vi "Dark Current Test Remastered Test Run.vi"() -> ()   [LabVIEW 2020]
uses:
  <vilib>/Utility/file.llb/Write Delimited Spreadsheet (string).vi
  <vilib>/Utility/file.llb/Write Delimited Spreadsheet (DBL).vi
  <instrlib>/CAEN PSM/CAEN PSM.lvlib
panel:
  out "7 4":bool
  out "6 4":bool
  out "8 4":bool
  out "5 4":bool
  out "4 4":bool
  out "3 4":bool
  out "2 4":bool
  out "1 4":bool
  out "Test is Running 4":bool
  out "OVV? 8":bool=TRUE
  out "OVC? 8":bool=TRUE
  out "Actual Voltage Level (V) 8":dbl format="%#_13g"
  out "Actual Current Limit (nA) 4":dbl format="%#_13g"
  in  "dt (s) 4":i32
  out "Time Left (s) 4":dbl
  out "Power Supply Trip 4":bool
  in  "N 4":i32
  in  "Channel # 4":i32
  in  "VISA resource name 4":refnum<visa-resource-name>
  out "OVV? 7":bool=TRUE
  out "OVC? 7":bool=TRUE
  out "Actual Voltage Level (V) 7":dbl format="%#_13g"
  out "Recorded Current\nfor Previous Tube 4":dbl format="%#_13g"
  in  "Measure Next Tube 4":bool
  out "Next Measurment 4":string
  in  "Barcodes 4":string[](array[string])
  out "Manual Measurments \nNeeded 4":bool
  in  "Begin Test 4":bool
  out "7 3":bool
  out "6 3":bool
  out "8 3":bool
  out "5 3":bool
  out "4 3":bool
  out "3 3":bool
  out "2 3":bool
  out "1 3":bool
  out "Test is Running 3":bool
  out "OVV? 6":bool=TRUE
  out "OVC? 6":bool=TRUE
  out "Actual Voltage Level (V) 6":dbl format="%#_13g"
  out "Actual Current Limit (nA) 3":dbl format="%#_13g"
  in  "dt (s) 3":i32
  out "Time Left (s) 3":dbl
  out "Power Supply Trip 3":bool
  in  "N 3":i32
  in  "Channel # 3":i32
  in  "VISA resource name 3":refnum<visa-resource-name>
  out "OVV? 5":bool=TRUE
  out "OVC? 5":bool=TRUE
  out "Actual Voltage Level (V) 5":dbl format="%#_13g"
  out "Recorded Current\nfor Previous Tube 3":dbl format="%#_13g"
  in  "Measure Next Tube 3":bool
  out "Next Measurment 3":string
  in  "Barcodes 3":string[](array[string])
  out "Manual Measurments \nNeeded 3":bool
  in  "Begin Test 3":bool
  out "7 2":bool
  out "6 2":bool
  out "8 2":bool
  out "5 2":bool
  out "4 2":bool
  out "3 2":bool
  out "2 2":bool
  out "1 2":bool
  out "Test is Running 2":bool
  out "OVV? 4":bool=TRUE
  out "OVC? 4":bool=TRUE
  out "Actual Voltage Level (V) 4":dbl format="%#_13g"
  out "Actual Current Limit (nA) 2":dbl format="%#_13g"
  in  "dt (s) 2":i32
  out "Time Left (s) 2":dbl
  out "Power Supply Trip 2":bool
  in  "N 2":i32
  in  "Channel # 2":i32
  in  "VISA resource name 2":refnum<visa-resource-name>
  out "OVV? 3":bool=TRUE
  out "OVC? 3":bool=TRUE
  out "Actual Voltage Level (V) 3":dbl format="%#_13g"
  out "Recorded Current\nfor Previous Tube 2":dbl format="%#_13g"
  in  "Measure Next Tube 2":bool
  out "Next Measurment 2":string
  in  "Barcodes 2":string[](array[string])
  out "Manual Measurments \nNeeded 2":bool
  in  "Begin Test 2":bool
  out "Power Supply Trip":bool
  out "Time Left (s)":dbl
  out "8":bool
  out "7":bool
  out "6":bool
  out "5":bool
  out "4":bool
  out "3":bool
  out "2":bool
  out "1":bool
  out "Test is Running":bool
  in  "Begin Test":bool
  out "Manual Measurments \nNeeded":bool
  out "OVV? 2":bool=TRUE
  out "OVC? 2":bool=TRUE
  out "Actual Voltage Level (V) 2":dbl format="%#_13g"
  out "Recorded Current\nfor Previous Tube":dbl format="%#_13g"
  in  "Measure Next Tube":bool
  in  "Barcodes":string[](array[string])
  out "Next Measurment":string
  in  "N":i32
  in  "dt (s)":i32
  out "Actual Current Limit (nA)":dbl format="%#_13g"
  out "Actual Voltage Level (V)":dbl format="%#_13g"
  out "OVC?":bool=TRUE
  out "OVV?":bool=TRUE
  in  "Channel #":i32
  in  "VISA resource name":refnum<visa-resource-name>
  # "Dark Current Test"
  # "Instructions in Brief:\n1. Begin the program by clicking the white arrow.\n2. Assemble tubes into the test bench.\n3. Select COM5 for the \"VISA resource name\".\n4. Enter in how often you want to take measurement in the \"dt\" box (typically 60s)\n5. Enter in how many measurments you want to take (typically 15)\n6. Scan in the 8 tubes that you are testing.\n(If you take 15 measurments every 60s, the test will take 15 min.)\n7. Click \"Begin Test\". The \"Test is Running\" LED should light up.\n8. After the intial test, if the total current is below 16nA, \n    the program will write the \n     file and end the test.\n9. If the total current is above 16nA, manual\n    measurments need to be taken.\n10. Engage only the tube indicated by \"Next Measurment\". \n11. Click \"Measure\".\n12. Engage the next tube and continue untill all have been measured.\n13. In both cases, the program will write files and end the test. \n14. The test is over when the \"Test is Running\" LED has turned off."
  # "Green lights indicate tubes that have passed."
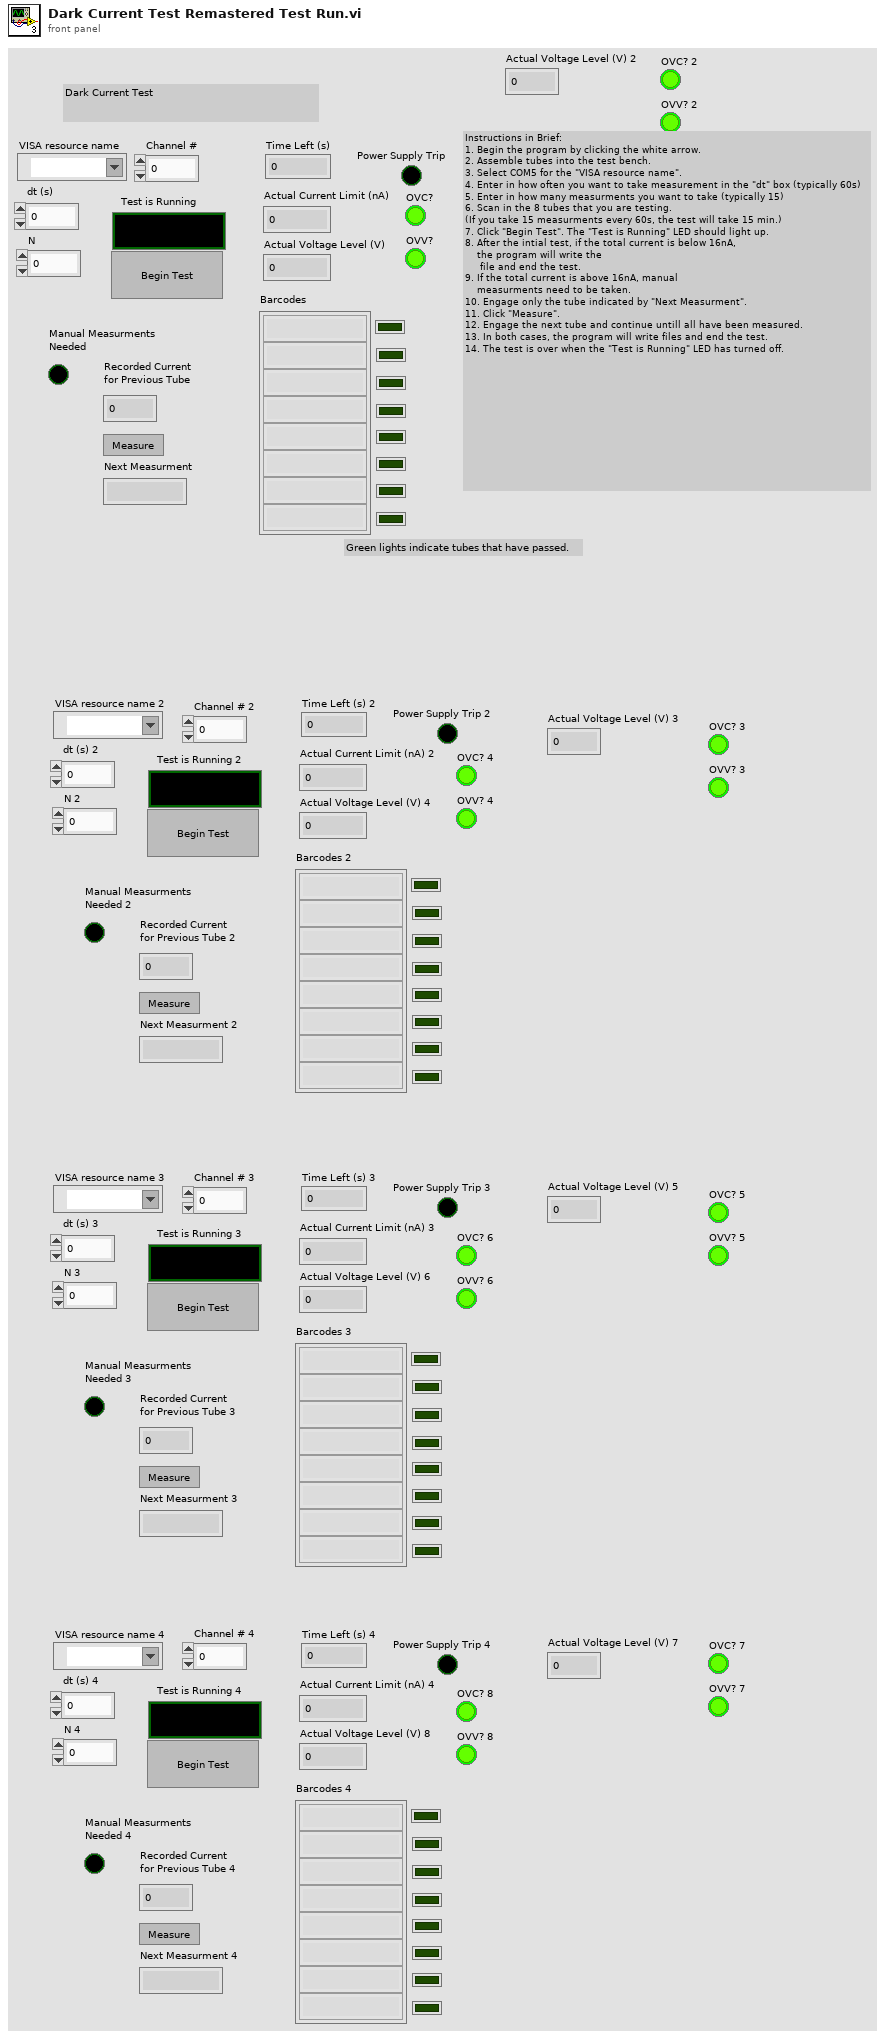
[diagram p1: front panel]
types:
  T1 = cluster{"VISA resource name":refnum<visa-resource-name>, "Board address":u8, "NChannels":u8}
  T2 = cluster{"ON":bool, "RUP":bool, "RDW":bool, "OVC":bool, "OVV":bool, "UNV":bool, "MAXV":bool, "TRIP":bool, "OVP":bool, "OVT":bool, "DIS":bool, "KILL":bool, "ILK":bool, "NOCAL":bool}[]
  T3 = cluster{"ON":bool, "RUP":bool, "RDW":bool, "OVC":bool, "OVV":bool, "UNV":bool, "MAXV":bool, "TRIP":bool, "OVP":bool, "OVT":bool, "DIS":bool, "KILL":bool, "ILK":bool, "NOCAL":bool}
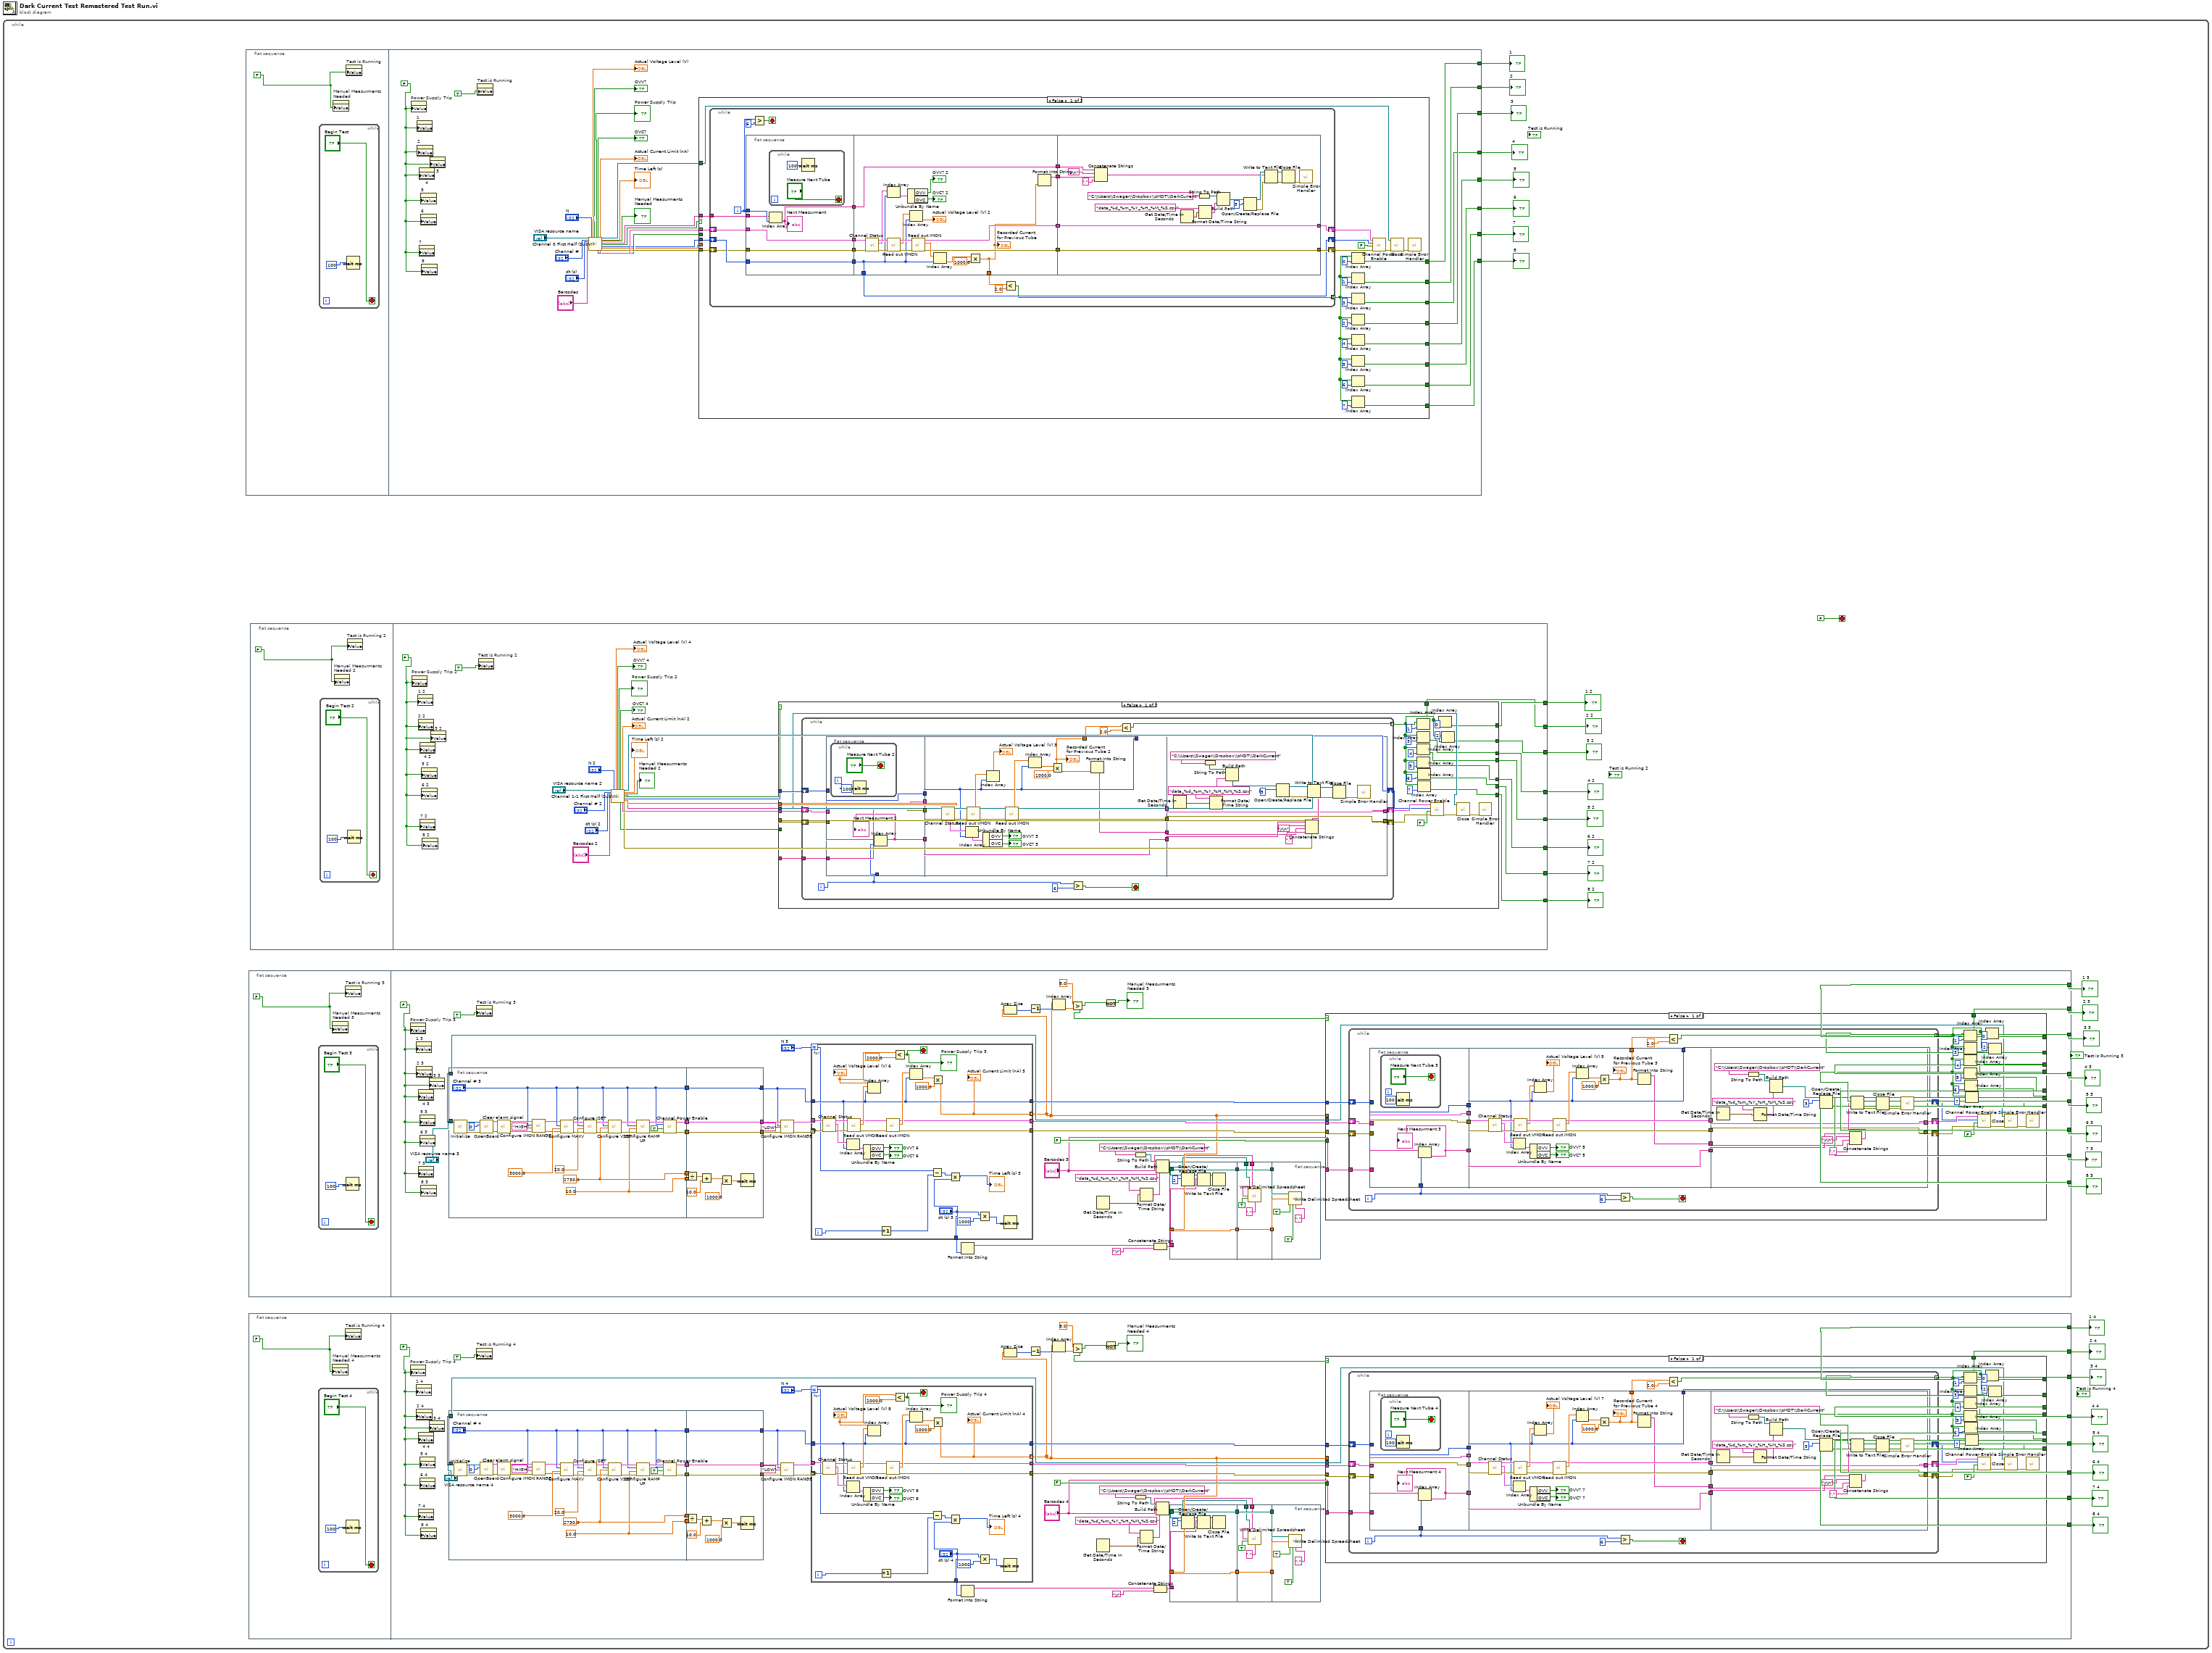
[diagram p0: block diagram]
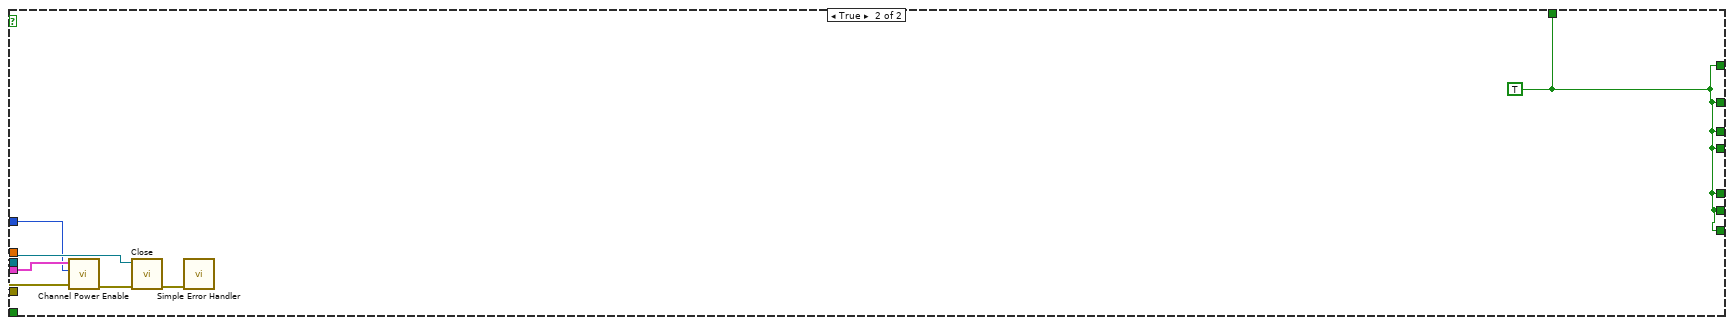
[diagram p2: hidden frame]
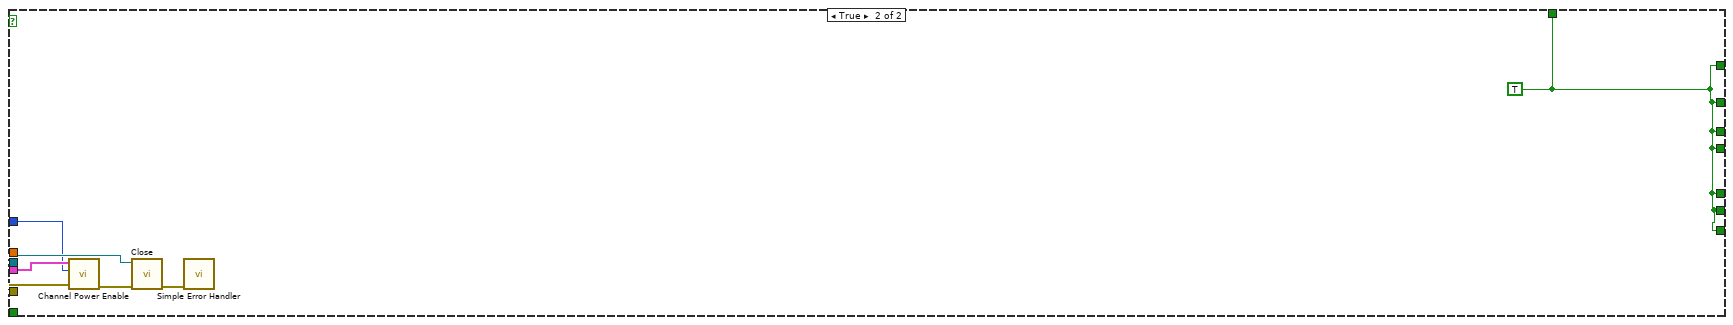
[diagram p3: hidden frame]
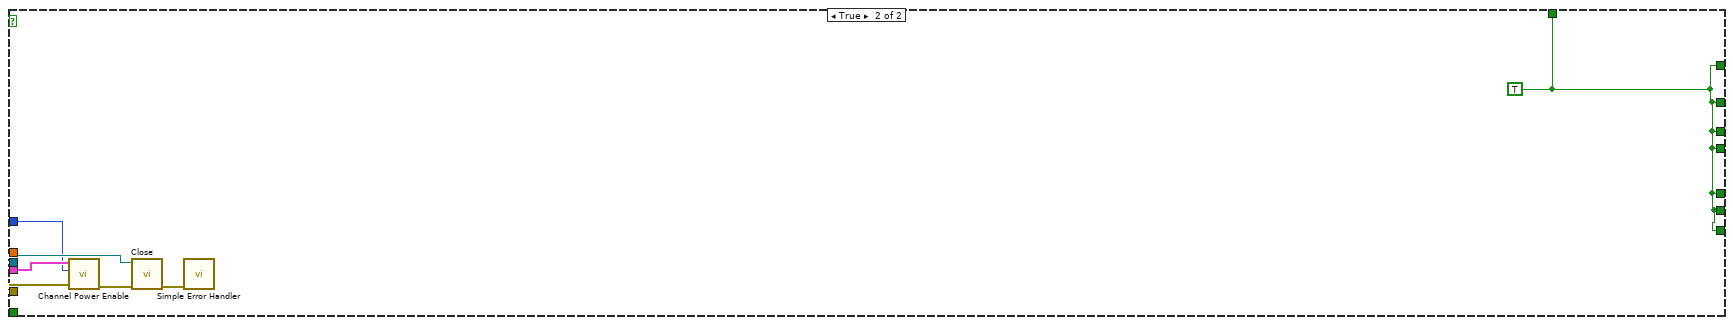
[diagram p4: hidden frame]
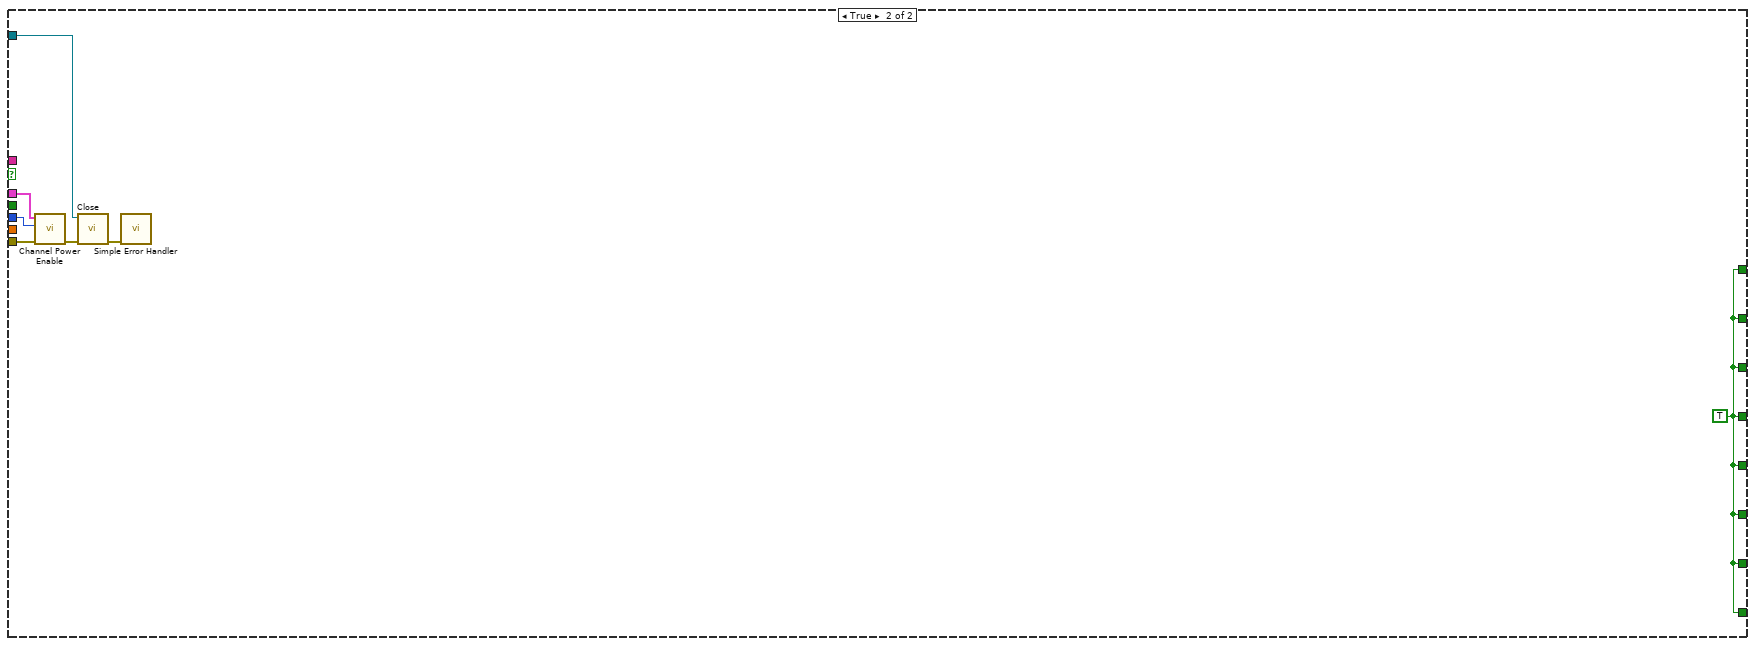
[diagram p5: hidden frame]
diagram:
  n1 = while {
    stop <- FALSE stop-if-true
    n2 = flat-sequence {
      tunnel: [w678] -> w32
      tunnel: [w658] -> w31
      tunnel: [w677] -> w30
      tunnel: [w676] -> w29
      tunnel: [w675] -> w28
      tunnel: [w659] -> w27
      tunnel: [w674] -> w26
      tunnel: [w673] -> w25
      frame #0 {
        w655 = FALSE
        n3 = while {
          stop <- "Begin Test" stop-if-true
          n4 = Wait (ms)(milliseconds to wait=100) -> ()  [unwired: 1 out]
        }
        n5 = property on="Manual Measurments \nNeeded" class="Bool (strict)"("Value"=w655) -> ()  [unwired: 2 in, 2 out]
        n6 = property on="Test is Running" class="Bool (strict)"("Value"=w655) -> ()  [unwired: 2 in, 2 out]
      }
      frame #1 {
        w671 = FALSE
        n7 = property on="Power Supply Trip" class="Bool (strict)"("Value"=w671) -> ()  [unwired: 2 in, 2 out]
        n8 = property on="1" class="Bool (strict)"("Value"=w671) -> ()  [unwired: 2 in, 2 out]
        n9 = property on="2" class="Bool (strict)"("Value"=w671) -> ()  [unwired: 2 in, 2 out]
        n10 = property on="4" class="Bool (strict)"("Value"=w671) -> ()  [unwired: 2 in, 2 out]
        n11 = property on="7" class="Bool (strict)"("Value"=w671) -> ()  [unwired: 2 in, 2 out]
        n12 = property on="5" class="Bool (strict)"("Value"=w671) -> ()  [unwired: 2 in, 2 out]
        n13 = property on="6" class="Bool (strict)"("Value"=w671) -> ()  [unwired: 2 in, 2 out]
        n14 = property on="8" class="Bool (strict)"("Value"=w671) -> ()  [unwired: 2 in, 2 out]
        n15 = property on="3" class="Bool (strict)"("Value"=w671) -> ()  [unwired: 2 in, 2 out]
        n16 = property on="Test is Running" class="Bool (strict)"("Value"=TRUE) -> ()  [unwired: 2 in, 2 out]
        n17 = call "Channel 0 First Half (SubVI).vi"("VISA Refnum in"="VISA resource name", "Channel #"="Channel #", "dt (s)"="dt (s)", "Barcodes in"="Barcodes", "N"="N") -> ("Actual Voltage Level (V)"=→"Actual Voltage Level (V)":dbl, "OVV?"=→"OVV?":bool, "Power Supply Trip"=→"Power Supply Trip":bool, "OVC?"=→"OVC?":bool, "Boolean 2"=w684:bool, "Actual Current Limit (nA)"=→"Actual Current Limit (nA)":dbl, "BoardHandle out 2"=w686:T1, "VISA Refnum out"=w682:refnum<visa-resource-name>, "Time Left (s)"=→"Time Left (s)":dbl, "Manual Measurments \nNeeded"=→"Manual Measurments \nNeeded":bool, "Barcodes out"=w670:string[], "Boolean"=w680:bool, "Channel # out 2"=w683:i32, "Array"=w672:dbl[], "error out"=w685:errorcluster)  [unwired: 8 in]
        n18 = case shown="False" w680 {
          tunnel: w686 -> [w714 w787]
          tunnel: w685 -> [w715 w786]
          tunnel: w684 -> [_ _]
          tunnel: w683 -> [w713 w785]
          tunnel: w682 -> [w709 w788]
          tunnel: w672 -> [_ _]
          tunnel: w670 -> [w705 _]
          tunnel: [w695 w791] -> w678
          tunnel: [w694 w791] -> w658
          tunnel: [w693 w791] -> w677
          tunnel: [w692 w791] -> w676
          tunnel: [w691 w791] -> w675
          tunnel: [w690 w791] -> w659
          tunnel: [w689 w791] -> w674
          tunnel: [w688 w791] -> w673
          frame False {
            n19 = while {
              shift-right: [w721] -> w706
              shift-left: w713 -> [w731]
              shift-right: [w723] -> w708
              shift-left: w714 -> [w728]
              shift-right: [w722] -> w707
              shift-left: w715 -> [w726]
              tunnel: w705 -> [w719]
              tunnel: [w716] -> w704 mode=indexing
              i -> [w734]
              stop <- w735 stop-if-true
              n20 = flat-sequence {
                tunnel: w734 -> [w742]
                tunnel: [w741] -> w733
                tunnel: w731 -> [w740]
                tunnel: [w740] -> w730
                tunnel: [w739] -> w729
                tunnel: w728 -> [w739]
                tunnel: [w738] -> w727
                tunnel: w726 -> [w738]
                tunnel: w719 -> [w737]
                tunnel: w733 -> [w752]
                tunnel: [w752] -> w732
                tunnel: w730 -> [w747]
                tunnel: w729 -> [w750]
                tunnel: w727 -> [w751]
                tunnel: [w749] -> w725
                tunnel: [w748] -> w724
                tunnel: [w747] -> w721
                tunnel: [w746] -> w720
                tunnel: [w745] -> w718
                tunnel: w732 -> [w770]
                tunnel: w725 -> [w768]
                tunnel: w724 -> [w767]
                tunnel: [w768] -> w723
                tunnel: [w767] -> w722
                tunnel: w720 -> [w766]
                frame #0 {
                  n21 = while {
                    stop <- "Measure Next Tube" stop-if-true
                    n22 = Wait (ms)(milliseconds to wait=100) -> ()  [unwired: 1 out]
                  }
                  n23 = Index Array(array=w737, index=w742) -> (element=w741:string)
                  "Next Measurment" <- w741
                }
                frame #1 {
                  n24 = call <instrlib>:"Channel Status.vi"("error in (no error)"=w751, "BoardHandle"=w750) -> ("error out"=w758:errorcluster, "Channel Status Array"=w754:T2, "BoardHandle out"=w759:T1)  [unwired: 7 in]
                  n25 = Index Array(array=w754, index=w747) -> (element=w755:T3)
                  n26 = call <instrlib>:"Read out VMON.vi"("error in (no error)"=w758, "BoardHandle"=w759) -> ("error out"=w762:errorcluster, "VMon values (V)"=w760:dbl[], "BoardHandle out"=w761:T1)  [unwired: 7 in]
                  n27 = Unbundle By Name(w755) -> ("OVV"=→"OVV? 2":bool, "OVC"=→"OVC? 2":bool)
                  n28 = Index Array(array=w760, index=w747) -> (element=→"Actual Voltage Level (V) 2":dbl)
                  n29 = call <instrlib>:"Read out IMON.vi"("error in (no error)"=w762, "BoardHandle"=w761) -> ("error out"=w748:errorcluster, "IMon values (uA)"=w765:dbl[], "BoardHandle out"=w749:T1)  [unwired: 6 in, 1 out]
                  n30 = Index Array(array=w765, index=w747) -> (element=w763:dbl)
                  n31 = Multiply(x=w763, y=1000.0) -> (x*y=w745:dbl)
                  "Recorded Current\nfor Previous Tube" <- w745
                  n32 = Format Into String(w745) -> (resulting string=w746:string)  [unwired: 3 in, 1 out]
                }
                frame #2 {
                  n33 = Concatenate Strings(w770, "\r\n", w766, ",") -> (w772:string)
                  n34 = Get Date/Time In Seconds() -> (seconds since 1Jan1904=w782:timestamp)
                  n35 = String To Path(string="C:\\Users\\Swager\\Dropbox\\sMDT\\DarkCurrent") -> (path=w781:path)
                  n36 = Format Date/Time String(time format string (%c)="data_%d_%m_%Y_%H_%M_%S.csv", seconds (now)=w782) -> (date/time string=w783:string)  [unwired: 1 in]
                  n37 = Build Path(base path=w781, name or relative path=w783) -> (appended path=w779:path)
                  n38 = Open/Create/Replace File(file path (use dialog)=w779, operation (0:open)=5) -> (refnum out=w778:refnum<file>, error out=w777:errorcluster)  [unwired: 4 in, 1 out]
                  n39 = Write to Text File(file (use dialog)=w778, text=w772, error in=w777) -> (refnum out=w776:refnum<file>, error out=w775:errorcluster)  [unwired: 1 in, 1 out]
                  n40 = Close File(refnum=w776, error in=w775) -> (error out=w774:errorcluster)  [unwired: 1 out]
                  n41 = call <vilib>:"Simple Error Handler.vi"("error in (no error)"=w774) -> ()  [unwired: 4 in, 5 out]
                }
              }
              n42 = Greater?(x=w734, y=6) -> (0:w735:bool)
              n43 = Less?(x=w718, y=2.0) -> (x < y?=w716:bool)
            }
            n44 = Index Array(array=w704, index=0) -> (element=w695:bool)
            n45 = Index Array(array=w704, index=1) -> (element=w694:bool)
            n46 = Index Array(array=w704, index=3) -> (element=w692:bool)
            n47 = Index Array(array=w704, index=2) -> (element=w693:bool)
            n48 = Index Array(array=w704, index=4) -> (element=w691:bool)
            n49 = Index Array(array=w704, index=5) -> (element=w690:bool)
            n50 = Index Array(array=w704, index=6) -> (element=w689:bool)
            n51 = Index Array(array=w704, index=7) -> (element=w688:bool)
            n52 = call <instrlib>:"Channel Power Enable.vi"("error in (no error)"=w707, "Enable (OFF)"=FALSE, "Channel (0)"=w706, "BoardHandle"=w708) -> ("error out"=w711:errorcluster)  [unwired: 6 in, 1 out]
            n53 = call <instrlib>:"Close.vi"("error in (no error)"=w711, "VISA resource name"=w709) -> ("error out"=w710:errorcluster)  [unwired: 9 in]
            n54 = call <vilib>:"Simple Error Handler.vi"("error in (no error)"=w710) -> ()  [unwired: 4 in, 5 out]
          }
          frame True {
            w791 = TRUE
            n55 = call <instrlib>:"Channel Power Enable.vi"("error in (no error)"=w786, "Channel (0)"=w785, "BoardHandle"=w787) -> ("error out"=w790:errorcluster)  [unwired: 7 in, 1 out]
            n56 = call <instrlib>:"Close.vi"("error in (no error)"=w790, "VISA resource name"=w788) -> ("error out"=w789:errorcluster)  [unwired: 9 in]
            n57 = call <vilib>:"Simple Error Handler.vi"("error in (no error)"=w789) -> ()  [unwired: 4 in, 5 out]
          }
        }
      }
    }
    n58 = flat-sequence {
      tunnel: [w303] -> w16
      tunnel: [w302] -> w15
      tunnel: [w301] -> w14
      tunnel: [w300] -> w13
      tunnel: [w299] -> w12
      tunnel: [w298] -> w11
      tunnel: [w297] -> w10
      tunnel: [w296] -> w9
      frame #0 {
        w276 = FALSE
        n59 = while {
          stop <- "Begin Test 3" stop-if-true
          n60 = Wait (ms)(milliseconds to wait=100) -> ()  [unwired: 1 out]
        }
        n61 = property on="Manual Measurments \nNeeded 3" class="Bool (strict)"("Value"=w276) -> ()  [unwired: 2 in, 2 out]
        n62 = property on="Test is Running 3" class="Bool (strict)"("Value"=w276) -> ()  [unwired: 2 in, 2 out]
      }
      frame #1 {
        w289 = FALSE
        n63 = property on="Power Supply Trip 3" class="Bool (strict)"("Value"=w289) -> ()  [unwired: 2 in, 2 out]
        n64 = property on="1 3" class="Bool (strict)"("Value"=w289) -> ()  [unwired: 2 in, 2 out]
        n65 = property on="2 3" class="Bool (strict)"("Value"=w289) -> ()  [unwired: 2 in, 2 out]
        n66 = property on="4 3" class="Bool (strict)"("Value"=w289) -> ()  [unwired: 2 in, 2 out]
        n67 = property on="7 3" class="Bool (strict)"("Value"=w289) -> ()  [unwired: 2 in, 2 out]
        n68 = property on="5 3" class="Bool (strict)"("Value"=w289) -> ()  [unwired: 2 in, 2 out]
        n69 = property on="6 3" class="Bool (strict)"("Value"=w289) -> ()  [unwired: 2 in, 2 out]
        n70 = property on="8 3" class="Bool (strict)"("Value"=w289) -> ()  [unwired: 2 in, 2 out]
        n71 = property on="3 3" class="Bool (strict)"("Value"=w289) -> ()  [unwired: 2 in, 2 out]
        n72 = flat-sequence {
          tunnel: [w463] -> w328
          tunnel: [w462] -> w327
          tunnel: [w459] -> w318
          tunnel: [w461] -> w326
          tunnel: [w460] -> w325
          tunnel: ["Channel # 3"] -> w324
          tunnel: "VISA resource name 3" -> [w459]
          tunnel: w328 -> [w483]
          tunnel: w327 -> [w482]
          tunnel: [w481] -> w315
          tunnel: w326 -> [w481]
          tunnel: [w480] -> w316
          tunnel: w325 -> [w480]
          tunnel: [w479] -> w313
          tunnel: w324 -> [w479]
          frame #0 {
            w463 = 2730.0 ("Voltage Set (Volts)")
            w462 = 10.0 ("Voltage Ramp Up (V/s)")
            n73 = call <instrlib>:"Initialize.vi"("VISA resource name"=w459) -> ("error out"=w473:errorcluster, "VISA resource name out"=w469:refnum<visa-resource-name>)  [unwired: 9 in]
            n74 = call <instrlib>:"OpenBoard.vi"("error in (no error)"=w473, "Board Address"=0, "VISA resource name"=w469) -> ("error out"=w474:errorcluster, "BoardHandle"=w468:T1)  [unwired: 7 in]
            n75 = call <instrlib>:"Clear alarm signal.vi"("error in (no error)"=w474, "BoardHandle"=w468) -> ("error out"=w457:errorcluster, "BoardHandle out"=w456:T1)  [unwired: 8 in]
            n76 = call <instrlib>:"Configure IMON RANGE.vi"("error in (no error)"=w457, "IMon range (LOW)"="HIGH", "Channel (0)"="Channel # 3", "BoardHandle"=w456) -> ("error out"=w452:errorcluster, "BoardHandle out"=w453:T1)  [unwired: 6 in]
            n77 = call <instrlib>:"Configure MAXV.vi"("error in (no error)"=w452, "Voltage Max (0.0 V)"=3000.0 ("VMax (Volts)"), "Channel (0)"="Channel # 3", "BoardHandle"=w453) -> ("error out"=w475:errorcluster, "BoardHandle out"=w467:T1)  [unwired: 6 in]
            n78 = call <instrlib>:"Configure ISET.vi"("error in (no error)"=w475, "Current Limit (0.00 uA)"=20.0 ("Current Limit (uA)"), "Channel (0)"="Channel # 3", "BoardHandle"=w467) -> ("error out"=w476:errorcluster, "BoardHandle out"=w466:T1)  [unwired: 6 in]
            n79 = call <instrlib>:"Configure VSET.vi"("error in (no error)"=w476, "Voltage Level (0.0 V)"=w463, "Channel (0)"="Channel # 3", "BoardHandle"=w466) -> ("error out"=w477:errorcluster, "BoardHandle out"=w465:T1)  [unwired: 6 in]
            n80 = call <instrlib>:"Configure RAMP UP.vi"("error in (no error)"=w477, "Voltage ramp up (0 V/s)"=w462, "Channel (0)"="Channel # 3", "BoardHandle"=w465) -> ("error out"=w478:errorcluster, "BoardHandle out"=w464:T1)  [unwired: 6 in]
            n81 = call <instrlib>:"Channel Power Enable.vi"("error in (no error)"=w478, "Enable (OFF)"=TRUE ("Boolean"), "Channel (0)"="Channel # 3", "BoardHandle"=w464) -> ("error out"=w460:errorcluster, "BoardHandle out"=w461:T1)  [unwired: 6 in]
          }
          frame #1 {
            n82 = Divide(x=w483, y=w482) -> (x/y=w486:dbl)
            n83 = Add(x=w486, y=10.0) -> (x+y=w487:dbl)
            n84 = Multiply(x=w487, y=1000.0) -> (x*y=w488:dbl)
            n85 = Wait (ms)(milliseconds to wait=w488) -> ()  [unwired: 1 out]
          }
        }
        n86 = property on="Test is Running 3" class="Bool (strict)"("Value"=TRUE) -> ()  [unwired: 2 in, 2 out]
        n87 = call <instrlib>:"Configure IMON RANGE.vi"("error in (no error)"=w316, "IMon range (LOW)"="LOW", "Channel (0)"=w313, "BoardHandle"=w315) -> ("error out"=w311:errorcluster, "BoardHandle out"=w312:T1)  [unwired: 6 in]
        n88 = for {
          N: "N 3" -> [w497]
          tunnel: w311 -> [w504]
          tunnel: w313 -> [w505]
          tunnel: [w507] -> w322
          tunnel: [w506] -> w321
          tunnel: [w498] -> w290 mode=indexing
          tunnel: [w505] -> w319
          tunnel: w312 -> [w501]
          tunnel: [w504] -> _ mode=indexing
          tunnel: ["dt (s) 3"] -> w288
          i -> [w494]
          stop <- w492 stop-if-true
          n89 = call <instrlib>:"Channel Status.vi"("error in (no error)"=w504, "BoardHandle"=w501) -> ("error out"=w513:errorcluster, "Channel Status Array"=w517:T2, "BoardHandle out"=w512:T1)  [unwired: 7 in]
          n90 = Index Array(array=w517, index=w505) -> (element=w516:T3)
          n91 = call <instrlib>:"Read out VMON.vi"("error in (no error)"=w513, "BoardHandle"=w512) -> ("error out"=w509:errorcluster, "VMon values (V)"=w511:dbl[], "BoardHandle out"=w510:T1)  [unwired: 7 in]
          n92 = Unbundle By Name(w516) -> ("OVV"=→"OVV? 6":bool, "OVC"=→"OVC? 6":bool)
          n93 = Index Array(array=w511, index=w505) -> (element=w491:dbl)
          "Actual Voltage Level (V) 6" <- w491
          n94 = Increment(x=w494) -> (x+1=w493:i32)
          n95 = call <instrlib>:"Read out IMON.vi"("error in (no error)"=w509, "BoardHandle"=w510) -> ("error out"=w506:errorcluster, "IMon values (uA)"=w508:dbl[], "BoardHandle out"=w507:T1)  [unwired: 6 in, 1 out]
          n96 = Less?(x=w491, y=2000.0) -> (x < y?=w492:bool)
          "Power Supply Trip 3" <- w492
          n97 = Index Array(array=w508, index=w505) -> (element=w500:dbl)
          n98 = Subtract(x=w497, y=w493) -> (x-y=w496:i32)
          n99 = Multiply(x=w500, y=1000.0) -> (x*y=w498:dbl)
          "Actual Current Limit (nA) 3" <- w498
          n100 = Multiply(x=w496, y="dt (s) 3") -> (x*y=→"Time Left (s) 3":i32)
          n101 = Multiply(x="dt (s) 3", y=1000) -> (x*y=w503:i32)
          n102 = Wait (ms)(milliseconds to wait=w503) -> ()  [unwired: 1 out]
        }
        n103 = Format Into String(w288) -> (resulting string=w280:string)  [unwired: 3 in, 1 out]
        n104 = Array Size(array=w290) -> (size(s)=w310:i32)
        n105 = Decrement(x=w310) -> (x-1=w309:i32)
        n106 = Index Array(array=w290, index=w309) -> (element=w308:dbl)
        n107 = Greater?(x=8.0, y=w308) -> (0:w307:bool)
        n108 = Get Date/Time In Seconds() -> (seconds since 1Jan1904=w293:timestamp)
        n109 = Not(x=w307) -> (.not. x?=→"Manual Measurments \nNeeded 3":bool)
        n110 = String To Path(string="C:\\Users\\Swager\\Dropbox\\sMDT\\DarkCurrent") -> (path=w292:path)
        n111 = Format Date/Time String(time format string (%c)="data_%d_%m_%Y_%H_%M_%S.csv", seconds (now)=w293) -> (date/time string=w294:string)  [unwired: 1 in]
        n112 = Concatenate Strings(w280, "\r") -> (w281:string)
        n113 = Build Path(base path=w292, name or relative path=w294) -> (appended path=w283:path)
        n114 = flat-sequence {
          tunnel: w283 -> [w335]
          tunnel: [w335] -> w287
          tunnel: [w336] -> w285
          tunnel: w290 -> [w336]
          tunnel: w281 -> [w332]
          tunnel: w287 -> [w342]
          tunnel: [w342] -> w286
          tunnel: w285 -> [w341]
          tunnel: [w341] -> w284
          tunnel: w283 -> [w340]
          tunnel: "Barcodes 3" -> [w339]
          tunnel: w286 -> [w345]
          tunnel: w284 -> [w344]
          frame #0 {
            n115 = Open/Create/Replace File(file path (use dialog)=w335, operation (0:open)=2) -> (refnum out=w333:refnum<file>, error out=w334:errorcluster)  [unwired: 4 in, 1 out]
            n116 = Write to Text File(file (use dialog)=w333, text=w332, error in=w334) -> (refnum out=w330:refnum<file>, error out=w331:errorcluster)  [unwired: 1 in, 1 out]
            n117 = Close File(refnum=w330, error in=w331) -> ()  [unwired: 2 out]
          }
          frame #1 {
            n118 = call-poly <vilib>:"Write Delimited Spreadsheet.vi"("file path (dialog if empty)"=w340, "1D data"=w339, "append to file? (new file:F)"=TRUE, "delimiter (\\t)"=",") -> ()  [unwired: 10 in, 2 out]
          }
          frame #2 {
            n119 = call-poly <vilib>:"Write Delimited Spreadsheet.vi"("file path (dialog if empty)"=w345, "1D data"=w344, "append to file? (new file:F)"=TRUE, "transpose? (no:F)"=TRUE, "delimiter (\\t)"=",") -> ()  [unwired: 9 in, 2 out]
          }
        }
        n120 = case shown="False" w307 {
          tunnel: w322 -> [w374 w447]
          tunnel: w321 -> [w375 w446]
          tunnel: FALSE -> [_ _]
          tunnel: w319 -> [w373 w445]
          tunnel: w318 -> [w369 w448]
          tunnel: w290 -> [_ _]
          tunnel: "Barcodes 3" -> [w365 _]
          tunnel: [w355 w451] -> w303
          tunnel: [w354 w451] -> w302
          tunnel: [w353 w451] -> w301
          tunnel: [w352 w451] -> w300
          tunnel: [w351 w451] -> w299
          tunnel: [w350 w451] -> w298
          tunnel: [w349 w451] -> w297
          tunnel: [w348 w451] -> w296
          frame False {
            n121 = while {
              shift-right: [w381] -> w366
              shift-left: w373 -> [w391]
              shift-right: [w383] -> w368
              shift-left: w374 -> [w388]
              shift-right: [w382] -> w367
              shift-left: w375 -> [w386]
              tunnel: w365 -> [w379]
              tunnel: [w376] -> w364 mode=indexing
              i -> [w394]
              stop <- w395 stop-if-true
              n122 = flat-sequence {
                tunnel: w394 -> [w402]
                tunnel: [w401] -> w393
                tunnel: w391 -> [w400]
                tunnel: [w400] -> w390
                tunnel: [w399] -> w389
                tunnel: w388 -> [w399]
                tunnel: [w398] -> w387
                tunnel: w386 -> [w398]
                tunnel: w379 -> [w397]
                tunnel: w393 -> [w412]
                tunnel: [w412] -> w392
                tunnel: w390 -> [w407]
                tunnel: w389 -> [w410]
                tunnel: w387 -> [w411]
                tunnel: [w409] -> w385
                tunnel: [w408] -> w384
                tunnel: [w407] -> w381
                tunnel: [w406] -> w380
                tunnel: [w405] -> w378
                tunnel: w392 -> [w430]
                tunnel: w385 -> [w428]
                tunnel: w384 -> [w427]
                tunnel: [w428] -> w383
                tunnel: [w427] -> w382
                tunnel: w380 -> [w426]
                frame #0 {
                  n123 = while {
                    stop <- "Measure Next Tube 3" stop-if-true
                    n124 = Wait (ms)(milliseconds to wait=100) -> ()  [unwired: 1 out]
                  }
                  n125 = Index Array(array=w397, index=w402) -> (element=w401:string)
                  "Next Measurment 3" <- w401
                }
                frame #1 {
                  n126 = call <instrlib>:"Channel Status.vi"("error in (no error)"=w411, "BoardHandle"=w410) -> ("error out"=w418:errorcluster, "Channel Status Array"=w414:T2, "BoardHandle out"=w419:T1)  [unwired: 7 in]
                  n127 = Index Array(array=w414, index=w407) -> (element=w415:T3)
                  n128 = call <instrlib>:"Read out VMON.vi"("error in (no error)"=w418, "BoardHandle"=w419) -> ("error out"=w422:errorcluster, "VMon values (V)"=w420:dbl[], "BoardHandle out"=w421:T1)  [unwired: 7 in]
                  n129 = Unbundle By Name(w415) -> ("OVV"=→"OVV? 5":bool, "OVC"=→"OVC? 5":bool)
                  n130 = Index Array(array=w420, index=w407) -> (element=→"Actual Voltage Level (V) 5":dbl)
                  n131 = call <instrlib>:"Read out IMON.vi"("error in (no error)"=w422, "BoardHandle"=w421) -> ("error out"=w408:errorcluster, "IMon values (uA)"=w425:dbl[], "BoardHandle out"=w409:T1)  [unwired: 6 in, 1 out]
                  n132 = Index Array(array=w425, index=w407) -> (element=w423:dbl)
                  n133 = Multiply(x=w423, y=1000.0) -> (x*y=w405:dbl)
                  "Recorded Current\nfor Previous Tube 3" <- w405
                  n134 = Format Into String(w405) -> (resulting string=w406:string)  [unwired: 3 in, 1 out]
                }
                frame #2 {
                  n135 = Get Date/Time In Seconds() -> (seconds since 1Jan1904=w442:timestamp)
                  n136 = String To Path(string="C:\\Users\\Swager\\Dropbox\\sMDT\\DarkCurrent") -> (path=w441:path)
                  n137 = Format Date/Time String(time format string (%c)="data_%d_%m_%Y_%H_%M_%S.csv", seconds (now)=w442) -> (date/time string=w443:string)  [unwired: 1 in]
                  n138 = Build Path(base path=w441, name or relative path=w443) -> (appended path=w439:path)
                  n139 = Open/Create/Replace File(file path (use dialog)=w439, operation (0:open)=5) -> (refnum out=w438:refnum<file>, error out=w437:errorcluster)  [unwired: 4 in, 1 out]
                  n140 = Concatenate Strings(w430, "\r\n", w426, ",") -> (w432:string)
                  n141 = Write to Text File(file (use dialog)=w438, text=w432, error in=w437) -> (refnum out=w436:refnum<file>, error out=w435:errorcluster)  [unwired: 1 in, 1 out]
                  n142 = Close File(refnum=w436, error in=w435) -> (error out=w434:errorcluster)  [unwired: 1 out]
                  n143 = call <vilib>:"Simple Error Handler.vi"("error in (no error)"=w434) -> ()  [unwired: 4 in, 5 out]
                }
              }
              n144 = Greater?(x=w394, y=6) -> (0:w395:bool)
              n145 = Less?(x=w378, y=2.0) -> (x < y?=w376:bool)
            }
            n146 = Index Array(array=w364, index=1) -> (element=w354:bool)
            n147 = Index Array(array=w364, index=3) -> (element=w352:bool)
            n148 = Index Array(array=w364, index=4) -> (element=w351:bool)
            n149 = Index Array(array=w364, index=5) -> (element=w350:bool)
            n150 = Index Array(array=w364, index=6) -> (element=w349:bool)
            n151 = Index Array(array=w364, index=7) -> (element=w348:bool)
            n152 = call <instrlib>:"Channel Power Enable.vi"("error in (no error)"=w367, "Enable (OFF)"=FALSE, "Channel (0)"=w366, "BoardHandle"=w368) -> ("error out"=w371:errorcluster)  [unwired: 6 in, 1 out]
            n153 = Index Array(array=w364, index=0) -> (element=w355:bool)
            n154 = Index Array(array=w364, index=2) -> (element=w353:bool)
            n155 = call <instrlib>:"Close.vi"("error in (no error)"=w371, "VISA resource name"=w369) -> ("error out"=w370:errorcluster)  [unwired: 9 in]
            n156 = call <vilib>:"Simple Error Handler.vi"("error in (no error)"=w370) -> ()  [unwired: 4 in, 5 out]
          }
          frame True {
            w451 = TRUE
            n157 = call <instrlib>:"Channel Power Enable.vi"("error in (no error)"=w446, "Channel (0)"=w445, "BoardHandle"=w447) -> ("error out"=w450:errorcluster)  [unwired: 7 in, 1 out]
            n158 = call <instrlib>:"Close.vi"("error in (no error)"=w450, "VISA resource name"=w448) -> ("error out"=w449:errorcluster)  [unwired: 9 in]
            n159 = call <vilib>:"Simple Error Handler.vi"("error in (no error)"=w449) -> ()  [unwired: 4 in, 5 out]
          }
        }
      }
    }
    n160 = flat-sequence {
      tunnel: [w61] -> w8
      tunnel: [w60] -> w7
      tunnel: [w59] -> w6
      tunnel: [w58] -> w5
      tunnel: [w57] -> w4
      tunnel: [w56] -> w3
      tunnel: [w55] -> w2
      tunnel: [w54] -> w1
      frame #0 {
        w34 = FALSE
        n161 = while {
          stop <- "Begin Test 4" stop-if-true
          n162 = Wait (ms)(milliseconds to wait=100) -> ()  [unwired: 1 out]
        }
        n163 = property on="Manual Measurments \nNeeded 4" class="Bool (strict)"("Value"=w34) -> ()  [unwired: 2 in, 2 out]
        n164 = property on="Test is Running 4" class="Bool (strict)"("Value"=w34) -> ()  [unwired: 2 in, 2 out]
      }
      frame #1 {
        w47 = FALSE
        n165 = property on="Power Supply Trip 4" class="Bool (strict)"("Value"=w47) -> ()  [unwired: 2 in, 2 out]
        n166 = property on="1 4" class="Bool (strict)"("Value"=w47) -> ()  [unwired: 2 in, 2 out]
        n167 = property on="2 4" class="Bool (strict)"("Value"=w47) -> ()  [unwired: 2 in, 2 out]
        n168 = property on="4 4" class="Bool (strict)"("Value"=w47) -> ()  [unwired: 2 in, 2 out]
        n169 = property on="7 4" class="Bool (strict)"("Value"=w47) -> ()  [unwired: 2 in, 2 out]
        n170 = property on="5 4" class="Bool (strict)"("Value"=w47) -> ()  [unwired: 2 in, 2 out]
        n171 = property on="6 4" class="Bool (strict)"("Value"=w47) -> ()  [unwired: 2 in, 2 out]
        n172 = property on="8 4" class="Bool (strict)"("Value"=w47) -> ()  [unwired: 2 in, 2 out]
        n173 = property on="3 4" class="Bool (strict)"("Value"=w47) -> ()  [unwired: 2 in, 2 out]
        n174 = flat-sequence {
          tunnel: [w221] -> w86
          tunnel: [w220] -> w85
          tunnel: [w217] -> w76
          tunnel: [w219] -> w84
          tunnel: [w218] -> w83
          tunnel: ["Channel # 4"] -> w82
          tunnel: "VISA resource name 4" -> [w217]
          tunnel: w86 -> [w241]
          tunnel: w85 -> [w240]
          tunnel: [w239] -> w73
          tunnel: w84 -> [w239]
          tunnel: [w238] -> w74
          tunnel: w83 -> [w238]
          tunnel: [w237] -> w71
          tunnel: w82 -> [w237]
          frame #0 {
            w221 = 2730.0 ("Voltage Set (Volts)")
            w220 = 10.0 ("Voltage Ramp Up (V/s)")
            n175 = call <instrlib>:"Initialize.vi"("VISA resource name"=w217) -> ("error out"=w231:errorcluster, "VISA resource name out"=w227:refnum<visa-resource-name>)  [unwired: 9 in]
            n176 = call <instrlib>:"OpenBoard.vi"("error in (no error)"=w231, "Board Address"=0, "VISA resource name"=w227) -> ("error out"=w232:errorcluster, "BoardHandle"=w226:T1)  [unwired: 7 in]
            n177 = call <instrlib>:"Clear alarm signal.vi"("error in (no error)"=w232, "BoardHandle"=w226) -> ("error out"=w215:errorcluster, "BoardHandle out"=w214:T1)  [unwired: 8 in]
            n178 = call <instrlib>:"Configure IMON RANGE.vi"("error in (no error)"=w215, "IMon range (LOW)"="HIGH", "Channel (0)"="Channel # 4", "BoardHandle"=w214) -> ("error out"=w210:errorcluster, "BoardHandle out"=w211:T1)  [unwired: 6 in]
            n179 = call <instrlib>:"Configure MAXV.vi"("error in (no error)"=w210, "Voltage Max (0.0 V)"=3000.0 ("VMax (Volts)"), "Channel (0)"="Channel # 4", "BoardHandle"=w211) -> ("error out"=w233:errorcluster, "BoardHandle out"=w225:T1)  [unwired: 6 in]
            n180 = call <instrlib>:"Configure ISET.vi"("error in (no error)"=w233, "Current Limit (0.00 uA)"=20.0 ("Current Limit (uA)"), "Channel (0)"="Channel # 4", "BoardHandle"=w225) -> ("error out"=w234:errorcluster, "BoardHandle out"=w224:T1)  [unwired: 6 in]
            n181 = call <instrlib>:"Configure VSET.vi"("error in (no error)"=w234, "Voltage Level (0.0 V)"=w221, "Channel (0)"="Channel # 4", "BoardHandle"=w224) -> ("error out"=w235:errorcluster, "BoardHandle out"=w223:T1)  [unwired: 6 in]
            n182 = call <instrlib>:"Configure RAMP UP.vi"("error in (no error)"=w235, "Voltage ramp up (0 V/s)"=w220, "Channel (0)"="Channel # 4", "BoardHandle"=w223) -> ("error out"=w236:errorcluster, "BoardHandle out"=w222:T1)  [unwired: 6 in]
            n183 = call <instrlib>:"Channel Power Enable.vi"("error in (no error)"=w236, "Enable (OFF)"=TRUE ("Boolean"), "Channel (0)"="Channel # 4", "BoardHandle"=w222) -> ("error out"=w218:errorcluster, "BoardHandle out"=w219:T1)  [unwired: 6 in]
          }
          frame #1 {
            n184 = Divide(x=w241, y=w240) -> (x/y=w244:dbl)
            n185 = Add(x=w244, y=10.0) -> (x+y=w245:dbl)
            n186 = Multiply(x=w245, y=1000.0) -> (x*y=w246:dbl)
            n187 = Wait (ms)(milliseconds to wait=w246) -> ()  [unwired: 1 out]
          }
        }
        n188 = property on="Test is Running 4" class="Bool (strict)"("Value"=TRUE) -> ()  [unwired: 2 in, 2 out]
        n189 = call <instrlib>:"Configure IMON RANGE.vi"("error in (no error)"=w74, "IMon range (LOW)"="LOW", "Channel (0)"=w71, "BoardHandle"=w73) -> ("error out"=w69:errorcluster, "BoardHandle out"=w70:T1)  [unwired: 6 in]
        n190 = for {
          N: "N 4" -> [w255]
          tunnel: w69 -> [w262]
          tunnel: w71 -> [w263]
          tunnel: [w265] -> w80
          tunnel: [w264] -> w79
          tunnel: [w256] -> w48 mode=indexing
          tunnel: [w263] -> w77
          tunnel: w70 -> [w259]
          tunnel: [w262] -> _ mode=indexing
          tunnel: ["dt (s) 4"] -> w46
          i -> [w252]
          stop <- w250 stop-if-true
          n191 = call <instrlib>:"Channel Status.vi"("error in (no error)"=w262, "BoardHandle"=w259) -> ("error out"=w271:errorcluster, "Channel Status Array"=w275:T2, "BoardHandle out"=w270:T1)  [unwired: 7 in]
          n192 = Index Array(array=w275, index=w263) -> (element=w274:T3)
          n193 = call <instrlib>:"Read out VMON.vi"("error in (no error)"=w271, "BoardHandle"=w270) -> ("error out"=w267:errorcluster, "VMon values (V)"=w269:dbl[], "BoardHandle out"=w268:T1)  [unwired: 7 in]
          n194 = Unbundle By Name(w274) -> ("OVV"=→"OVV? 8":bool, "OVC"=→"OVC? 8":bool)
          n195 = Index Array(array=w269, index=w263) -> (element=w249:dbl)
          "Actual Voltage Level (V) 8" <- w249
          n196 = Increment(x=w252) -> (x+1=w251:i32)
          n197 = call <instrlib>:"Read out IMON.vi"("error in (no error)"=w267, "BoardHandle"=w268) -> ("error out"=w264:errorcluster, "IMon values (uA)"=w266:dbl[], "BoardHandle out"=w265:T1)  [unwired: 6 in, 1 out]
          n198 = Less?(x=w249, y=2000.0) -> (x < y?=w250:bool)
          "Power Supply Trip 4" <- w250
          n199 = Index Array(array=w266, index=w263) -> (element=w258:dbl)
          n200 = Subtract(x=w255, y=w251) -> (x-y=w254:i32)
          n201 = Multiply(x=w258, y=1000.0) -> (x*y=w256:dbl)
          "Actual Current Limit (nA) 4" <- w256
          n202 = Multiply(x=w254, y="dt (s) 4") -> (x*y=→"Time Left (s) 4":i32)
          n203 = Multiply(x="dt (s) 4", y=1000) -> (x*y=w261:i32)
          n204 = Wait (ms)(milliseconds to wait=w261) -> ()  [unwired: 1 out]
        }
        n205 = Format Into String(w46) -> (resulting string=w38:string)  [unwired: 3 in, 1 out]
        n206 = Array Size(array=w48) -> (size(s)=w68:i32)
        n207 = Decrement(x=w68) -> (x-1=w67:i32)
        n208 = Index Array(array=w48, index=w67) -> (element=w66:dbl)
        n209 = Greater?(x=8.0, y=w66) -> (0:w65:bool)
        n210 = Get Date/Time In Seconds() -> (seconds since 1Jan1904=w51:timestamp)
        n211 = Not(x=w65) -> (.not. x?=→"Manual Measurments \nNeeded 4":bool)
        n212 = String To Path(string="C:\\Users\\Swager\\Dropbox\\sMDT\\DarkCurrent") -> (path=w50:path)
        n213 = Format Date/Time String(time format string (%c)="data_%d_%m_%Y_%H_%M_%S.csv", seconds (now)=w51) -> (date/time string=w52:string)  [unwired: 1 in]
        n214 = Concatenate Strings(w38, "\r") -> (w39:string)
        n215 = Build Path(base path=w50, name or relative path=w52) -> (appended path=w41:path)
        n216 = flat-sequence {
          tunnel: w41 -> [w93]
          tunnel: [w93] -> w45
          tunnel: [w94] -> w43
          tunnel: w48 -> [w94]
          tunnel: w39 -> [w90]
          tunnel: w45 -> [w100]
          tunnel: [w100] -> w44
          tunnel: w43 -> [w99]
          tunnel: [w99] -> w42
          tunnel: w41 -> [w98]
          tunnel: "Barcodes 4" -> [w97]
          tunnel: w44 -> [w103]
          tunnel: w42 -> [w102]
          frame #0 {
            n217 = Open/Create/Replace File(file path (use dialog)=w93, operation (0:open)=2) -> (refnum out=w91:refnum<file>, error out=w92:errorcluster)  [unwired: 4 in, 1 out]
            n218 = Write to Text File(file (use dialog)=w91, text=w90, error in=w92) -> (refnum out=w88:refnum<file>, error out=w89:errorcluster)  [unwired: 1 in, 1 out]
            n219 = Close File(refnum=w88, error in=w89) -> ()  [unwired: 2 out]
          }
          frame #1 {
            n220 = call-poly <vilib>:"Write Delimited Spreadsheet.vi"("file path (dialog if empty)"=w98, "1D data"=w97, "append to file? (new file:F)"=TRUE, "delimiter (\\t)"=",") -> ()  [unwired: 10 in, 2 out]
          }
          frame #2 {
            n221 = call-poly <vilib>:"Write Delimited Spreadsheet.vi"("file path (dialog if empty)"=w103, "1D data"=w102, "append to file? (new file:F)"=TRUE, "transpose? (no:F)"=TRUE, "delimiter (\\t)"=",") -> ()  [unwired: 9 in, 2 out]
          }
        }
        n222 = case shown="False" w65 {
          tunnel: w80 -> [w132 w205]
          tunnel: w79 -> [w133 w204]
          tunnel: FALSE -> [_ _]
          tunnel: w77 -> [w131 w203]
          tunnel: w76 -> [w127 w206]
          tunnel: w48 -> [_ _]
          tunnel: "Barcodes 4" -> [w123 _]
          tunnel: [w113 w209] -> w61
          tunnel: [w112 w209] -> w60
          tunnel: [w111 w209] -> w59
          tunnel: [w110 w209] -> w58
          tunnel: [w109 w209] -> w57
          tunnel: [w108 w209] -> w56
          tunnel: [w107 w209] -> w55
          tunnel: [w106 w209] -> w54
          frame False {
            n223 = while {
              shift-right: [w139] -> w124
              shift-left: w131 -> [w149]
              shift-right: [w141] -> w126
              shift-left: w132 -> [w146]
              shift-right: [w140] -> w125
              shift-left: w133 -> [w144]
              tunnel: w123 -> [w137]
              tunnel: [w134] -> w122 mode=indexing
              i -> [w152]
              stop <- w153 stop-if-true
              n224 = flat-sequence {
                tunnel: w152 -> [w160]
                tunnel: [w159] -> w151
                tunnel: w149 -> [w158]
                tunnel: [w158] -> w148
                tunnel: [w157] -> w147
                tunnel: w146 -> [w157]
                tunnel: [w156] -> w145
                tunnel: w144 -> [w156]
                tunnel: w137 -> [w155]
                tunnel: w151 -> [w170]
                tunnel: [w170] -> w150
                tunnel: w148 -> [w165]
                tunnel: w147 -> [w168]
                tunnel: w145 -> [w169]
                tunnel: [w167] -> w143
                tunnel: [w166] -> w142
                tunnel: [w165] -> w139
                tunnel: [w164] -> w138
                tunnel: [w163] -> w136
                tunnel: w150 -> [w188]
                tunnel: w143 -> [w186]
                tunnel: w142 -> [w185]
                tunnel: [w186] -> w141
                tunnel: [w185] -> w140
                tunnel: w138 -> [w184]
                frame #0 {
                  n225 = while {
                    stop <- "Measure Next Tube 4" stop-if-true
                    n226 = Wait (ms)(milliseconds to wait=100) -> ()  [unwired: 1 out]
                  }
                  n227 = Index Array(array=w155, index=w160) -> (element=w159:string)
                  "Next Measurment 4" <- w159
                }
                frame #1 {
                  n228 = call <instrlib>:"Channel Status.vi"("error in (no error)"=w169, "BoardHandle"=w168) -> ("error out"=w176:errorcluster, "Channel Status Array"=w172:T2, "BoardHandle out"=w177:T1)  [unwired: 7 in]
                  n229 = Index Array(array=w172, index=w165) -> (element=w173:T3)
                  n230 = call <instrlib>:"Read out VMON.vi"("error in (no error)"=w176, "BoardHandle"=w177) -> ("error out"=w180:errorcluster, "VMon values (V)"=w178:dbl[], "BoardHandle out"=w179:T1)  [unwired: 7 in]
                  n231 = Unbundle By Name(w173) -> ("OVV"=→"OVV? 7":bool, "OVC"=→"OVC? 7":bool)
                  n232 = Index Array(array=w178, index=w165) -> (element=→"Actual Voltage Level (V) 7":dbl)
                  n233 = call <instrlib>:"Read out IMON.vi"("error in (no error)"=w180, "BoardHandle"=w179) -> ("error out"=w166:errorcluster, "IMon values (uA)"=w183:dbl[], "BoardHandle out"=w167:T1)  [unwired: 6 in, 1 out]
                  n234 = Index Array(array=w183, index=w165) -> (element=w181:dbl)
                  n235 = Multiply(x=w181, y=1000.0) -> (x*y=w163:dbl)
                  "Recorded Current\nfor Previous Tube 4" <- w163
                  n236 = Format Into String(w163) -> (resulting string=w164:string)  [unwired: 3 in, 1 out]
                }
                frame #2 {
                  n237 = Get Date/Time In Seconds() -> (seconds since 1Jan1904=w200:timestamp)
                  n238 = String To Path(string="C:\\Users\\Swager\\Dropbox\\sMDT\\DarkCurrent") -> (path=w199:path)
                  n239 = Format Date/Time String(time format string (%c)="data_%d_%m_%Y_%H_%M_%S.csv", seconds (now)=w200) -> (date/time string=w201:string)  [unwired: 1 in]
                  n240 = Build Path(base path=w199, name or relative path=w201) -> (appended path=w197:path)
                  n241 = Open/Create/Replace File(file path (use dialog)=w197, operation (0:open)=5) -> (refnum out=w196:refnum<file>, error out=w195:errorcluster)  [unwired: 4 in, 1 out]
                  n242 = Concatenate Strings(w188, "\r\n", w184, ",") -> (w190:string)
                  n243 = Write to Text File(file (use dialog)=w196, text=w190, error in=w195) -> (refnum out=w194:refnum<file>, error out=w193:errorcluster)  [unwired: 1 in, 1 out]
                  n244 = Close File(refnum=w194, error in=w193) -> (error out=w192:errorcluster)  [unwired: 1 out]
                  n245 = call <vilib>:"Simple Error Handler.vi"("error in (no error)"=w192) -> ()  [unwired: 4 in, 5 out]
                }
              }
              n246 = Greater?(x=w152, y=6) -> (0:w153:bool)
              n247 = Less?(x=w136, y=2.0) -> (x < y?=w134:bool)
            }
            n248 = Index Array(array=w122, index=1) -> (element=w112:bool)
            n249 = Index Array(array=w122, index=3) -> (element=w110:bool)
            n250 = Index Array(array=w122, index=4) -> (element=w109:bool)
            n251 = Index Array(array=w122, index=5) -> (element=w108:bool)
            n252 = Index Array(array=w122, index=6) -> (element=w107:bool)
            n253 = Index Array(array=w122, index=7) -> (element=w106:bool)
            n254 = call <instrlib>:"Channel Power Enable.vi"("error in (no error)"=w125, "Enable (OFF)"=FALSE, "Channel (0)"=w124, "BoardHandle"=w126) -> ("error out"=w129:errorcluster)  [unwired: 6 in, 1 out]
            n255 = Index Array(array=w122, index=0) -> (element=w113:bool)
            n256 = Index Array(array=w122, index=2) -> (element=w111:bool)
            n257 = call <instrlib>:"Close.vi"("error in (no error)"=w129, "VISA resource name"=w127) -> ("error out"=w128:errorcluster)  [unwired: 9 in]
            n258 = call <vilib>:"Simple Error Handler.vi"("error in (no error)"=w128) -> ()  [unwired: 4 in, 5 out]
          }
          frame True {
            w209 = TRUE
            n259 = call <instrlib>:"Channel Power Enable.vi"("error in (no error)"=w204, "Channel (0)"=w203, "BoardHandle"=w205) -> ("error out"=w208:errorcluster)  [unwired: 7 in, 1 out]
            n260 = call <instrlib>:"Close.vi"("error in (no error)"=w208, "VISA resource name"=w206) -> ("error out"=w207:errorcluster)  [unwired: 9 in]
            n261 = call <vilib>:"Simple Error Handler.vi"("error in (no error)"=w207) -> ()  [unwired: 4 in, 5 out]
          }
        }
      }
    }
    n262 = flat-sequence {
      tunnel: [w541] -> w24
      tunnel: [w540] -> w23
      tunnel: [w539] -> w22
      tunnel: [w538] -> w21
      tunnel: [w537] -> w20
      tunnel: [w536] -> w19
      tunnel: [w535] -> w18
      tunnel: [w534] -> w17
      frame #0 {
        w518 = FALSE
        n263 = while {
          stop <- "Begin Test 2" stop-if-true
          n264 = Wait (ms)(milliseconds to wait=100) -> ()  [unwired: 1 out]
        }
        n265 = property on="Manual Measurments \nNeeded 2" class="Bool (strict)"("Value"=w518) -> ()  [unwired: 2 in, 2 out]
        n266 = property on="Test is Running 2" class="Bool (strict)"("Value"=w518) -> ()  [unwired: 2 in, 2 out]
      }
      frame #1 {
        w532 = FALSE
        n267 = property on="Power Supply Trip 2" class="Bool (strict)"("Value"=w532) -> ()  [unwired: 2 in, 2 out]
        n268 = property on="1 2" class="Bool (strict)"("Value"=w532) -> ()  [unwired: 2 in, 2 out]
        n269 = property on="2 2" class="Bool (strict)"("Value"=w532) -> ()  [unwired: 2 in, 2 out]
        n270 = property on="4 2" class="Bool (strict)"("Value"=w532) -> ()  [unwired: 2 in, 2 out]
        n271 = property on="7 2" class="Bool (strict)"("Value"=w532) -> ()  [unwired: 2 in, 2 out]
        n272 = property on="5 2" class="Bool (strict)"("Value"=w532) -> ()  [unwired: 2 in, 2 out]
        n273 = property on="6 2" class="Bool (strict)"("Value"=w532) -> ()  [unwired: 2 in, 2 out]
        n274 = property on="8 2" class="Bool (strict)"("Value"=w532) -> ()  [unwired: 2 in, 2 out]
        n275 = property on="3 2" class="Bool (strict)"("Value"=w532) -> ()  [unwired: 2 in, 2 out]
        n276 = property on="Test is Running 2" class="Bool (strict)"("Value"=TRUE) -> ()  [unwired: 2 in, 2 out]
        n277 = call "Channel 1-1 First Half (SubVI).vi"("VISA Refnum in"="VISA resource name 2", "Channel # in"="Channel # 2", "dt (s) in"="dt (s) 2", "Barcodes in"="Barcodes 2", "N in"="N 2") -> ("Actual Voltage Level (V) 4"=→"Actual Voltage Level (V) 4":dbl, "OVV? 4"=→"OVV? 4":bool, "Power Supply Trip 2"=→"Power Supply Trip 2":bool, "OVC? 4"=→"OVC? 4":bool, "Boolean 2"=w547:bool, "Actual Current Limit (nA) 2"=→"Actual Current Limit (nA) 2":dbl, "BoardHandle out 2"=w549:T1, "VISA Refnum out"=w545:refnum<visa-resource-name>, "Time Left (s) 2"=→"Time Left (s) 2":dbl, "Manual Measurments \nNeeded 2"=→"Manual Measurments \nNeeded 2":bool, "Barcodes 3"=w531:string[], "Boolean"=w543:bool, "Channel # 4"=w546:i32, "Array"=w533:dbl[], "error out"=w548:errorcluster)  [unwired: 8 in]
        n278 = case shown="False" w543 {
          tunnel: w549 -> [w577 w650]
          tunnel: w548 -> [w578 w649]
          tunnel: w547 -> [_ _]
          tunnel: w546 -> [w576 w648]
          tunnel: w545 -> [w572 w651]
          tunnel: w533 -> [_ _]
          tunnel: w531 -> [w568 _]
          tunnel: [w558 w654] -> w541
          tunnel: [w557 w654] -> w540
          tunnel: [w556 w654] -> w539
          tunnel: [w555 w654] -> w538
          tunnel: [w554 w654] -> w537
          tunnel: [w553 w654] -> w536
          tunnel: [w552 w654] -> w535
          tunnel: [w551 w654] -> w534
          frame False {
            n279 = while {
              shift-right: [w584] -> w569
              shift-left: w576 -> [w594]
              shift-right: [w586] -> w571
              shift-left: w577 -> [w591]
              shift-right: [w585] -> w570
              shift-left: w578 -> [w589]
              tunnel: w568 -> [w582]
              tunnel: [w579] -> w567 mode=indexing
              i -> [w597]
              stop <- w598 stop-if-true
              n280 = flat-sequence {
                tunnel: w597 -> [w605]
                tunnel: [w604] -> w596
                tunnel: w594 -> [w603]
                tunnel: [w603] -> w593
                tunnel: [w602] -> w592
                tunnel: w591 -> [w602]
                tunnel: [w601] -> w590
                tunnel: w589 -> [w601]
                tunnel: w582 -> [w600]
                tunnel: w596 -> [w615]
                tunnel: [w615] -> w595
                tunnel: w593 -> [w610]
                tunnel: w592 -> [w613]
                tunnel: w590 -> [w614]
                tunnel: [w612] -> w588
                tunnel: [w611] -> w587
                tunnel: [w610] -> w584
                tunnel: [w609] -> w583
                tunnel: [w608] -> w581
                tunnel: w595 -> [w633]
                tunnel: w588 -> [w631]
                tunnel: w587 -> [w630]
                tunnel: [w631] -> w586
                tunnel: [w630] -> w585
                tunnel: w583 -> [w629]
                frame #0 {
                  n281 = while {
                    stop <- "Measure Next Tube 2" stop-if-true
                    n282 = Wait (ms)(milliseconds to wait=100) -> ()  [unwired: 1 out]
                  }
                  n283 = Index Array(array=w600, index=w605) -> (element=w604:string)
                  "Next Measurment 2" <- w604
                }
                frame #1 {
                  n284 = call <instrlib>:"Channel Status.vi"("error in (no error)"=w614, "BoardHandle"=w613) -> ("error out"=w621:errorcluster, "Channel Status Array"=w617:T2, "BoardHandle out"=w622:T1)  [unwired: 7 in]
                  n285 = Index Array(array=w617, index=w610) -> (element=w618:T3)
                  n286 = call <instrlib>:"Read out VMON.vi"("error in (no error)"=w621, "BoardHandle"=w622) -> ("error out"=w625:errorcluster, "VMon values (V)"=w623:dbl[], "BoardHandle out"=w624:T1)  [unwired: 7 in]
                  n287 = Unbundle By Name(w618) -> ("OVV"=→"OVV? 3":bool, "OVC"=→"OVC? 3":bool)
                  n288 = Index Array(array=w623, index=w610) -> (element=→"Actual Voltage Level (V) 3":dbl)
                  n289 = call <instrlib>:"Read out IMON.vi"("error in (no error)"=w625, "BoardHandle"=w624) -> ("error out"=w611:errorcluster, "IMon values (uA)"=w628:dbl[], "BoardHandle out"=w612:T1)  [unwired: 6 in, 1 out]
                  n290 = Index Array(array=w628, index=w610) -> (element=w626:dbl)
                  n291 = Multiply(x=w626, y=1000.0) -> (x*y=w608:dbl)
                  "Recorded Current\nfor Previous Tube 2" <- w608
                  n292 = Format Into String(w608) -> (resulting string=w609:string)  [unwired: 3 in, 1 out]
                }
                frame #2 {
                  n293 = Get Date/Time In Seconds() -> (seconds since 1Jan1904=w645:timestamp)
                  n294 = String To Path(string="C:\\Users\\Swager\\Dropbox\\sMDT\\DarkCurrent") -> (path=w644:path)
                  n295 = Format Date/Time String(time format string (%c)="data_%d_%m_%Y_%H_%M_%S.csv", seconds (now)=w645) -> (date/time string=w646:string)  [unwired: 1 in]
                  n296 = Build Path(base path=w644, name or relative path=w646) -> (appended path=w642:path)
                  n297 = Open/Create/Replace File(file path (use dialog)=w642, operation (0:open)=5) -> (refnum out=w641:refnum<file>, error out=w640:errorcluster)  [unwired: 4 in, 1 out]
                  n298 = Concatenate Strings(w633, "\r\n", w629, ",") -> (w635:string)
                  n299 = Write to Text File(file (use dialog)=w641, text=w635, error in=w640) -> (refnum out=w639:refnum<file>, error out=w638:errorcluster)  [unwired: 1 in, 1 out]
                  n300 = Close File(refnum=w639, error in=w638) -> (error out=w637:errorcluster)  [unwired: 1 out]
                  n301 = call <vilib>:"Simple Error Handler.vi"("error in (no error)"=w637) -> ()  [unwired: 4 in, 5 out]
                }
              }
              n302 = Greater?(x=w597, y=6) -> (0:w598:bool)
              n303 = Less?(x=w581, y=2.0) -> (x < y?=w579:bool)
            }
            n304 = Index Array(array=w567, index=1) -> (element=w557:bool)
            n305 = Index Array(array=w567, index=3) -> (element=w555:bool)
            n306 = Index Array(array=w567, index=4) -> (element=w554:bool)
            n307 = Index Array(array=w567, index=5) -> (element=w553:bool)
            n308 = Index Array(array=w567, index=6) -> (element=w552:bool)
            n309 = Index Array(array=w567, index=7) -> (element=w551:bool)
            n310 = call <instrlib>:"Channel Power Enable.vi"("error in (no error)"=w570, "Enable (OFF)"=FALSE, "Channel (0)"=w569, "BoardHandle"=w571) -> ("error out"=w574:errorcluster)  [unwired: 6 in, 1 out]
            n311 = Index Array(array=w567, index=0) -> (element=w558:bool)
            n312 = Index Array(array=w567, index=2) -> (element=w556:bool)
            n313 = call <instrlib>:"Close.vi"("error in (no error)"=w574, "VISA resource name"=w572) -> ("error out"=w573:errorcluster)  [unwired: 9 in]
            n314 = call <vilib>:"Simple Error Handler.vi"("error in (no error)"=w573) -> ()  [unwired: 4 in, 5 out]
          }
          frame True {
            w654 = TRUE
            n315 = call <instrlib>:"Channel Power Enable.vi"("error in (no error)"=w649, "Channel (0)"=w648, "BoardHandle"=w650) -> ("error out"=w653:errorcluster)  [unwired: 7 in, 1 out]
            n316 = call <instrlib>:"Close.vi"("error in (no error)"=w653, "VISA resource name"=w651) -> ("error out"=w652:errorcluster)  [unwired: 9 in]
            n317 = call <vilib>:"Simple Error Handler.vi"("error in (no error)"=w652) -> ()  [unwired: 4 in, 5 out]
          }
        }
      }
    }
    "1" <- w32
    "2" <- w31
    "3" <- w30
    "4" <- w29
    "5" <- w28
    "8" <- w25
    "6" <- w27
    "7" <- w26
    "1 2" <- w24
    "2 2" <- w23
    "3 2" <- w22
    "4 2" <- w21
    "5 2" <- w20
    "8 2" <- w17
    "6 2" <- w19
    "7 2" <- w18
    "1 3" <- w16
    "2 3" <- w15
    "3 3" <- w14
    "4 3" <- w13
    "5 3" <- w12
    "8 3" <- w9
    "6 3" <- w11
    "7 3" <- w10
    "1 4" <- w8
    "2 4" <- w7
    "3 4" <- w6
    "4 4" <- w5
    "5 4" <- w4
    "8 4" <- w1
    "6 4" <- w3
    "7 4" <- w2
  }
